vi "Read PRACH Modulation Extreme Results.vi"(8 "error in (no error)":errorcluster, 10 "Instance (1)":T1=1, 11 "VISA resource name":refnum<visa-resource-name>) -> (0 "error out":errorcluster, 1 "Out Of Tolerance":i32, 2 "Reliability":i32, 3 "VISA resource name out":refnum<visa-resource-name>, 4 "Results":dbl[](array[numeric]) format="%^.3e")   [LabVIEW 2020, in "Rohde&Schwarz CMWXP NR FR1 Measurement.lvlib"]
doc: "Starts a new single shot measurement and returns the extreme single value modulation results.\n\nAttribute:\nRSCMWXPNRFR1M_ATTR_READ_PRACH_MODULATION_EXTREME_RESULTS\n\nRemote-control command:\nREAD:NRSub:MEAS<i>:PRACh:MODulation:EXTReme?"
uses:
  <instrlib>/Rohde&Schwarz CMWXP NR FR1 Measurement/Rohde&Schwarz CMWXP NR FR1 Measurement.lvlib
  <instrlib>/Rohde&Schwarz CMWXP NR FR1 Measurement/Private/_Instance.ctl
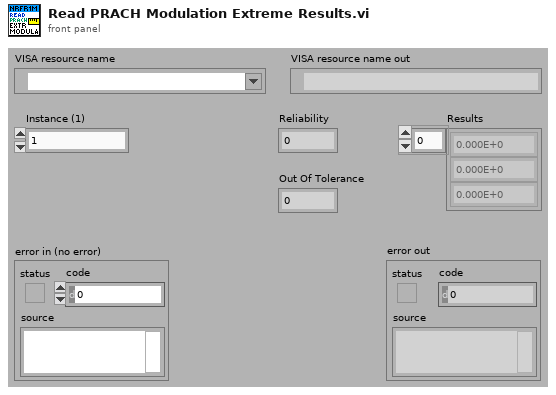
[diagram p1: front panel]
types:
  T1 = typedef "Rohde&Schwarz CMWXP NR FR1 Measurement.lvlib/_Instance.ctl" = i32
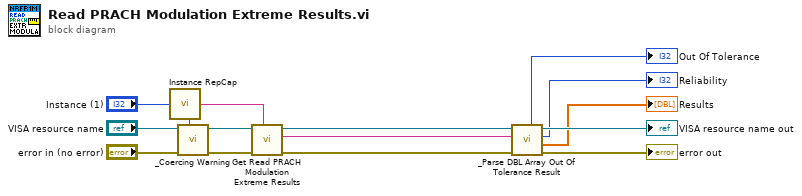
[diagram p0: block diagram]
diagram:
  n1 = call <instrlib>:"Instance RepCap.vi"("Instance In"="Instance (1)") -> ("In Range?"=w11:bool, "RepCap Identifier Out"=w9:string)  [unwired: 1 in]
  n2 = call <instrlib>:"_Coercing Warning.vi"("In Range?"=w11, "error in (no error)"="error in (no error)", "VISA resource name"="VISA resource name") -> ("error out"=w13:errorcluster, "VISA resource name out"=w12:refnum<visa-resource-name>)  [unwired: 7 in]
  n3 = call "Get Read PRACH Modulation Extreme Results"("Repeated Capabilities"=w9, "error in (no error)"=w13, "instrument handle"=w12) -> ("error out"=w8:errorcluster, "Read PRACH Modulation Extreme Results"=w4:string, "instrument handle out"=w5:refnum<visa-resource-name>)  [unwired: 6 in]
  n4 = call <instrlib>:"_Parse DBL Array Out Of Tolerance Result.vi"("error in (no error)"=w8, "Input String"=w4, "VISA resource name"=w5) -> ("error out"=→"error out":errorcluster, "Results"=→"Results":dbl[], "Reliability"=→"Reliability":i32, "VISA resource name out"=→"VISA resource name out":refnum<visa-resource-name>, "Out Of Tolerance"=→"Out Of Tolerance":i32)  [unwired: 4 in]
